vi "Get Folder Names.vi"(11 "Parent Tag":refnum<class "UTF-8 String.lvclass">) -> (3 "Folder Names":refnum<class "UTF-8 String.lvclass">[](array[class]))   [LabVIEW 2020, in "Tree Browser.lvlib"]
doc: "Gets the folder listing for a given parent tag (parent path). If parent tag is _ROOT_, returns a list of available disks (C:\\, D:\\, etc)."
uses:
  Tree Browser.lvlib
  Types/UTF-8 String/UTF-8 String.lvclass
  Types/UTF-8 String/UTF-8 String.lvclass/UTF-8 String.ctl
  Types/UTF-8 Path/UTF-8 Path.lvclass/UTF-8 Path.ctl
  6db467ac-ec2f-481a-b578-9c24b6b6728f.vi
  675e153a-17c1-44aa-829d-34786e782b4f.vi
  02f6871d-e7f4-4b3d-8634-939f7aca7cf7.vi
  8df487ab-a4e3-43cd-8a5c-f9e7e0a9aee7.vi
  792378cd-7439-4206-99b9-4938e13476f6.vi
  f6a40077-74b0-4618-a471-07fc7385b3d3.vi
  Private/Conversion/Text as Encoded Path.vi
  Private/Conversion/Polymorphic VIs/Text as Encoded Path (UTF-8 String).vi
  Types/UTF-8 Path/Write Encoded UTF-8 Path.vi
  Types/UTF-8 String/Write Encoded UTF-8 String.vi
  Private/Conversion/Path as UTF-8 Path.vi
  Private/Conversion/Polymorphic VIs/Path as UTF-8 Path (UTF-8 Path).vi
  675e153a-17c1-44aa-829d-34786e782b4f.vi/5269e09c-4216-478e-8686-9fb7d38e224a.vi
  675e153a-17c1-44aa-829d-34786e782b4f.vi/d1f4a45d-6f02-44dd-a40b-2b28d80e6519.vi
  Private/Conversion/String as Encoded String.vi
  Private/Conversion/Polymorphic VIs/String as Encoded String (UTF-8 String).vi
  Private/Library/gu_list_folder.vi
  675e153a-17c1-44aa-829d-34786e782b4f.vi/8eb4f0ed-0012-4550-978e-be3f7301df70.vi
  675e153a-17c1-44aa-829d-34786e782b4f.vi/f7e6584c-01ed-423f-9bcd-660954191d0d.vi
  Private/Conversion/Path as Encoded Path.vi
  Private/Conversion/Polymorphic VIs/Path as Encoded Path (UTF-8 Path).vi
  Private/Conversion/Text as Encoded String.vi
  Private/Conversion/Polymorphic VIs/Text as Encoded String (UTF-8 Path).vi
  Private/Conversion/Polymorphic VIs/Path as UTF-8 Path (LabVIEW Path).vi
  792378cd-7439-4206-99b9-4938e13476f6.vi/5269e09c-4216-478e-8686-9fb7d38e224a.vi
  792378cd-7439-4206-99b9-4938e13476f6.vi/d1f4a45d-6f02-44dd-a40b-2b28d80e6519.vi
  792378cd-7439-4206-99b9-4938e13476f6.vi/8eb4f0ed-0012-4550-978e-be3f7301df70.vi
  792378cd-7439-4206-99b9-4938e13476f6.vi/f7e6584c-01ed-423f-9bcd-660954191d0d.vi
  f6a40077-74b0-4618-a471-07fc7385b3d3.vi/b0de225b-b813-4a3f-91fa-b2c78c384815.vi
  f6a40077-74b0-4618-a471-07fc7385b3d3.vi/b1dd94da-e188-4359-85d0-d6693b26af46.vi
  f6a40077-74b0-4618-a471-07fc7385b3d3.vi/2799960a-efad-449d-b375-cc5363f1c370.vi
  f6a40077-74b0-4618-a471-07fc7385b3d3.vi/2ed7adf8-1da0-426c-b32d-a1b4538e7e16.vi
  675e153a-17c1-44aa-829d-34786e782b4f.vi/5269e09c-4216-478e-8686-9fb7d38e224a.vi/c24c063b-f849-48a1-b323-238a063d7118.vi
  675e153a-17c1-44aa-829d-34786e782b4f.vi/5269e09c-4216-478e-8686-9fb7d38e224a.vi/a2fd6c11-d594-45c9-8624-1f0a1df69df3.vi
  675e153a-17c1-44aa-829d-34786e782b4f.vi/5269e09c-4216-478e-8686-9fb7d38e224a.vi/1fd3173e-d32e-42cb-8f0d-819132eb8e27.vi
  675e153a-17c1-44aa-829d-34786e782b4f.vi/5269e09c-4216-478e-8686-9fb7d38e224a.vi/bb7c39fc-ad8e-447d-bc50-468674bfb562.vi
  Private/Library/Result To Error.vi
  675e153a-17c1-44aa-829d-34786e782b4f.vi/8eb4f0ed-0012-4550-978e-be3f7301df70.vi/3a31b270-3bb6-4c58-a256-c5fcc2c98f09.vi
  675e153a-17c1-44aa-829d-34786e782b4f.vi/8eb4f0ed-0012-4550-978e-be3f7301df70.vi/0ec5df2d-ef9b-4f84-a6a8-ffcedd45c4dc.vi
  Private/Conversion/Text as String.vi
  Private/Conversion/Polymorphic VIs/Text as String (UTF-8 Path).vi
  Types/UTF-8 Path/Read Encoded UTF-8 Path.vi
  Types/UTF-8 Path/New UTF-8 Path.vi
  792378cd-7439-4206-99b9-4938e13476f6.vi/5269e09c-4216-478e-8686-9fb7d38e224a.vi/c24c063b-f849-48a1-b323-238a063d7118.vi
  792378cd-7439-4206-99b9-4938e13476f6.vi/5269e09c-4216-478e-8686-9fb7d38e224a.vi/a2fd6c11-d594-45c9-8624-1f0a1df69df3.vi
  792378cd-7439-4206-99b9-4938e13476f6.vi/5269e09c-4216-478e-8686-9fb7d38e224a.vi/1fd3173e-d32e-42cb-8f0d-819132eb8e27.vi
  792378cd-7439-4206-99b9-4938e13476f6.vi/5269e09c-4216-478e-8686-9fb7d38e224a.vi/bb7c39fc-ad8e-447d-bc50-468674bfb562.vi
  792378cd-7439-4206-99b9-4938e13476f6.vi/8eb4f0ed-0012-4550-978e-be3f7301df70.vi/3a31b270-3bb6-4c58-a256-c5fcc2c98f09.vi
  792378cd-7439-4206-99b9-4938e13476f6.vi/8eb4f0ed-0012-4550-978e-be3f7301df70.vi/0ec5df2d-ef9b-4f84-a6a8-ffcedd45c4dc.vi
  Private/Conversion/Polymorphic VIs/String as Encoded String (LabVIEW String).vi
  Private/Library/gu_string_subset.vi
  Private/Library/gu_to_lower_case.vi
  Private/Library/gu_search_split_string.vi
  Private/Conversion/Polymorphic VIs/Text as Encoded String (UTF-8 String).vi
  Private/Conversion/Polymorphic VIs/Text as Encoded String (LabVIEW String).vi
  Unicode/Encode String.vi
  Private/Conversion/Text to UTF-8.vi
  Private/Conversion/Polymorphic VIs/Text to UTF-8 (LabVIEW String).vi
  Private/Memory/Copy String.vi
  Private/Conversion/Encoded UTF-8 String to Encoded UTF-16LE String.vi
  Private/Conversion/UTF-8 to Text.vi
  Private/Conversion/Polymorphic VIs/UTF-8 to Text (LabVIEW String).vi
  Private/Conversion/Encoded UTF-16LE String to Encoded UTF-8 String.vi
  Unicode/Prepend BOM.vi
  Private/Memory/Copy String.vi/4d47babd-4a2d-4eb7-b91b-7e707d692665.vi
  Private/Library/gu_free.vi
  Unicode/SubVIs/Byte Order Marks.vi
  Unicode/Detect BOM.vi
  <vilib>/Utility/error.llb/Error Cluster From Error Code.vi
  Private/Memory/Copy String Array.vi
  File IO/Path to Short Name (Unicode).vi
  Unicode/Detect String Encoding.vi
  Types/UTF-8 Path/UTF-8 Path.lvclass
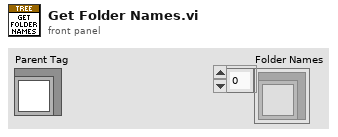
[diagram p1: front panel]
types:
  T1 = typedef "G-Unicode.lvlib/Encoded UTF-8 String.ctl" = string
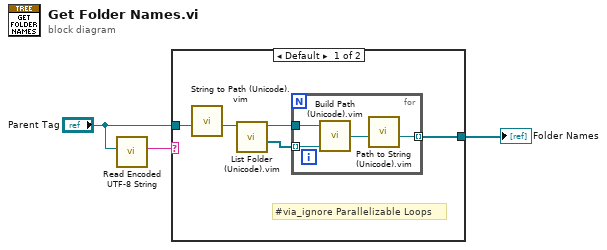
[diagram p0: block diagram]
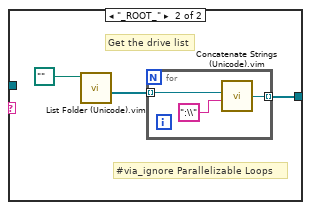
[diagram p2: hidden frame]
diagram:
  n1 = call "Read Encoded UTF-8 String.vi"("UTF-8 String"="Parent Tag") -> ("Encoded UTF-8 String"=w2:T1)  [unwired: 10 in]
  n2 = case shown="Default" w2 {
    tunnel: [w6 w13] -> w3
    tunnel: "Parent Tag" -> [w5 _]
    frame Default {
      # "#via_ignore Parallelizable Loops"
      n3 = call "String to Path (Unicode).vim"("String"=w5) -> ("Path"=w4:refnum<class "UTF-8 Path.lvclass">)  [unwired: 9 in, 1 out]
      n4 = call "List Folder (Unicode).vim"("Path"=w4) -> ("Folder Names"=w8:refnum<class "UTF-8 String.lvclass">[], "Path Out"=w7:refnum<class "UTF-8 Path.lvclass">)  [unwired: 7 in, 2 out]
      n5 = for {
        tunnel: w8 -> [w12] mode=indexing
        tunnel: w7 -> [w11]
        tunnel: [w10] -> w6 mode=indexing
        n6 = call "Build Path (Unicode).vim"("Base Path"=w11, "Name or Relative Path"=w12) -> ("Appended Path"=w9:refnum<class "UTF-8 Path.lvclass">)  [unwired: 6 in, 1 out]
        n7 = call "Path to String (Unicode).vim"("Path"=w9) -> ("String"=w10:refnum<class "UTF-8 String.lvclass">)  [unwired: 9 in, 1 out]
      }
    }
    frame "_ROOT_" {
      # "#via_ignore Parallelizable Loops"
      # "Get the drive list"
      n8 = call "List Folder (Unicode).vim"("Path"=path "") -> ("Folder Names"=w14:refnum<class "UTF-8 String.lvclass">[])  [unwired: 7 in, 3 out]
      n9 = for {
        tunnel: w14 -> [w17] mode=indexing
        tunnel: [w16] -> w13 mode=indexing
        n10 = call "Concatenate Strings (Unicode).vim"("Input 2"=":\\" ("string"), "Input 1"=w17) -> ("Concatenated String"=w16:refnum<class "UTF-8 String.lvclass">)  [unwired: 7 in, 1 out]
      }
    }
  }
  "Folder Names" <- w3
